vi "LOG Clear.vi"(8 "error in (no error)":errorcluster, 10 "Message Data":variant, 11 "Data Cluster":T1) -> (0 "error out":errorcluster, 3 "Data Cluster out":T1)   [LabVIEW 2020, in "LOG.lvlib"]
uses:
  LOG.lvlib
  LOG Configuration.ctl
  support/Message Queue/Message Cluster.ctl
  support/Message Queue/Message Queue.lvlib
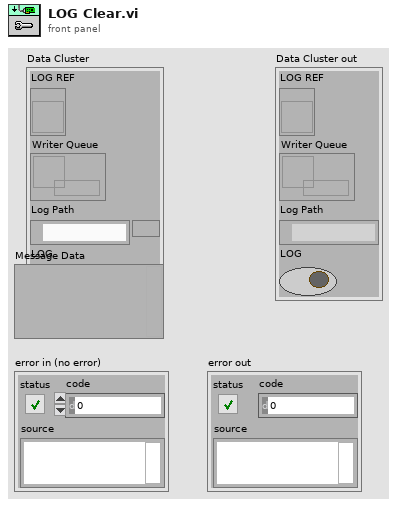
[diagram p1: front panel]
types:
  T1 = typedef "LOG.lvlib/LOG Configuration.ctl" = cluster{"LOG REF":refnum<vi>, "Writer Queue":refnum<queue>, "Log Path":path, "LOG":bool}
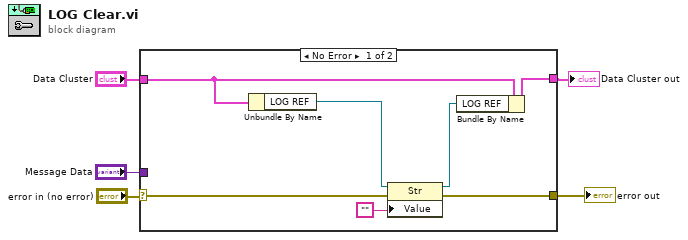
[diagram p0: block diagram]
diagram:
  n1 = case shown="No Error" "error in (no error)" {
    selector: "error in (no error)" -> [w7 w13]
    tunnel: [w12 w14] -> w4
    tunnel: "Data Cluster" -> [w11 w14]
    tunnel: [w10 w13] -> w3
    tunnel: "Message Data" -> [_ _]
    frame No Error {
      n2 = Unbundle By Name(w11) -> ("LOG REF"=w9:refnum<vi>)
      n3 = property class="Str"(reference=w9, error in=w7, "Value"="") -> (reference out=w8:refnum<vi>, error out=w10:errorcluster)
      n4 = Bundle By Name(cluster=w11, "LOG REF"=w8) -> (w12:T1)
    }
    frame Error {
    }
  }
  "error out" <- w3
  "Data Cluster out" <- w4
